vi "Freq-Mod.vi"() -> ()   [LabVIEW 2012]
uses:
  <vilib>/rvi/eio/common/nirviEmuTemplateMethod_errors.vi
  <vilib>/eio/EIONode/EIONode.xnode
panel:
  in  "Filter Constant":i16
  in  "Nominal Freq\nLIA":fxp<+/-,20,2>=0.20556640625 format="%#_9g"
  in  "K Constant":fxp<+/-,20,2>=1.52587890625e-05
  out "R(Amplitude)":i16
  in  "Sampling Frequency":i32=200000
  out "F Graph":i16
  in  "decimation":i16=1024
  in  "stages":i8=1
  in  "dec2":i16=1
  in  "dec1":i16=1
  out "Degrees":i16
  in  "phase setpoint":fxp<+/-,16,2>=1.57086181640625
  in  "alpha [U16.-2]":fxp<+,19,2>=0.01000213623046875
  in  "stop":bool
  out "sin(z) [I16.2]":fxp<+/-,16,2> format="%.15g"
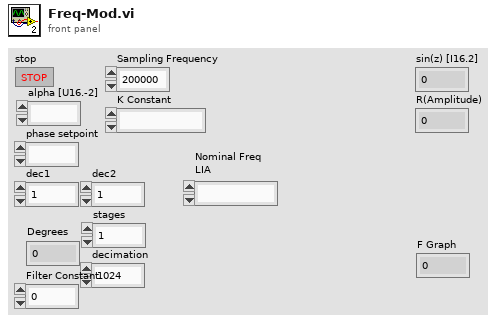
[diagram p1: front panel]
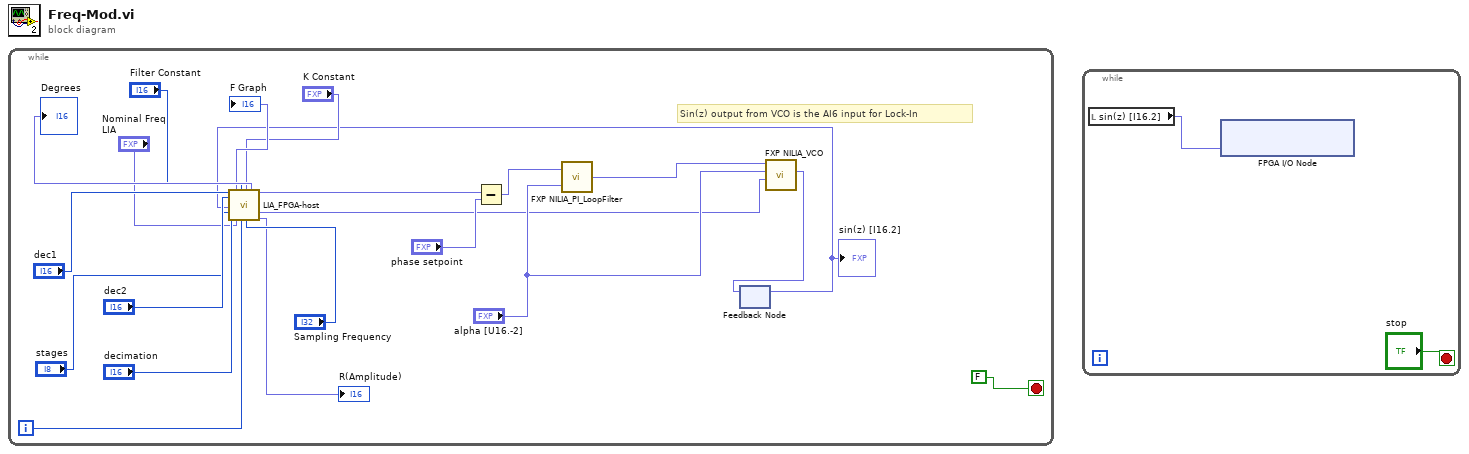
[diagram p0: block diagram]
diagram:
  n1 = while {
    i -> [w2]
    stop <- FALSE stop-if-true
    # "Sin(z) output from VCO is the AI6 input for Lock-In"
    n2 = feedback #1() -> (w3:fxp<+/-,16,2>)  [unwired: 1 in]
    "sin(z) [I16.2]" <- w3
    n3 = call "LIA_FPGA-host.vi"("dec1"="dec1", "dec2"="dec2", "Ref Signal"=w3, "stages"="stages", "decimation"="decimation", "nominal freq  (LIA)"="Nominal Freq\nLIA", "Filter Constant"="Filter Constant", "While Loop Counter"=w2, "K"="K Constant", "Sampling Frequency"="Sampling Frequency") -> ("F graph"=→"F Graph":fxp<+,64,64>, "Degree"=→"Degrees":fxp<+,1,1>, "phase (pi)"=w15:fxp<+/-,16,2>, "Nominal Freq"=w16:fxp<+/-,64,32>, "R"=→"R(Amplitude)":fxp<+,1,1>)  [unwired: 1 in, 4 out]
    n4 = Subtract(x=w15, y="phase setpoint") -> (x-y=w18:fxp<+/-,17,3>)
    n5 = call "FXP NILIA_PI_LoopFilter.vi"("alpha [U16.-2]"="alpha [U16.-2]", "x [I16.2]"=w18) -> ("x+y [I32.17]"=w21:fxp<+/-,32,17>)  [unwired: 1 in]
    n6 = call "FXP NILIA_VCO.vi"("nominal freq [U16.0]"=w16, "Kv [U16.0]"="alpha [U16.-2]", "v [I32.17]"=w21) -> ("sin(z) [I16.2]"=w4:fxp<+/-,16,2>)  [unwired: 5 in, 3 out]
    n7 = feedback-in #1(w4) -> ()
  }
  n8 = while {
    stop <- "stop" stop-if-true
    n9 = local read "sin(z) [I16.2]"() -> (w23:fxp<+/-,16,2>)
    n10 = xnode "FPGA I/O Node"("Connector0/AO5"=w23) -> ()  [unwired: 1 in, 1 out]
  }
